vi "Pomiar_UceIc.vi"(0 "Komutator L201":refnum<visa-resource-name>, 1 "Zasilacz BM572":refnum<visa-resource-name>, 2 "STOP":refnum<vi>, 5 "Samples":dbl[](array[numeric]), 9 "Multimetr V553":refnum<visa-resource-name>, 11 "Maksymalna moc tranzystora":dbl) -> (3 "Uce":dbl[](array[numeric]), 4 "Ic":dbl[](array[numeric]), 6 "Komutator L201 out":refnum<visa-resource-name>, 10 "Moc [W]":dbl[](array[numeric]), 12 "Multimetr V553 out":refnum<visa-resource-name>, 14 "Zasilacz BM572 out":refnum<visa-resource-name>, 15 "Index":i32)   [LabVIEW 2023]
panel:
  out "element":dbl
  out "String":string
  out "error constant 3":errorcluster
  out "error constant 2":errorcluster
  out "error constant":errorcluster
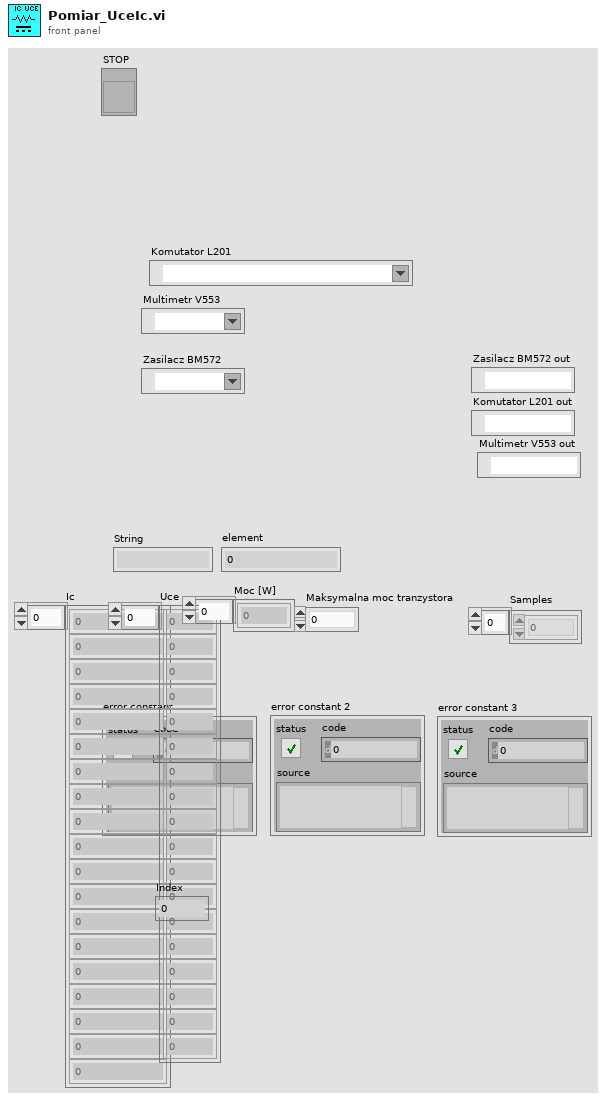
[diagram p1: front panel]
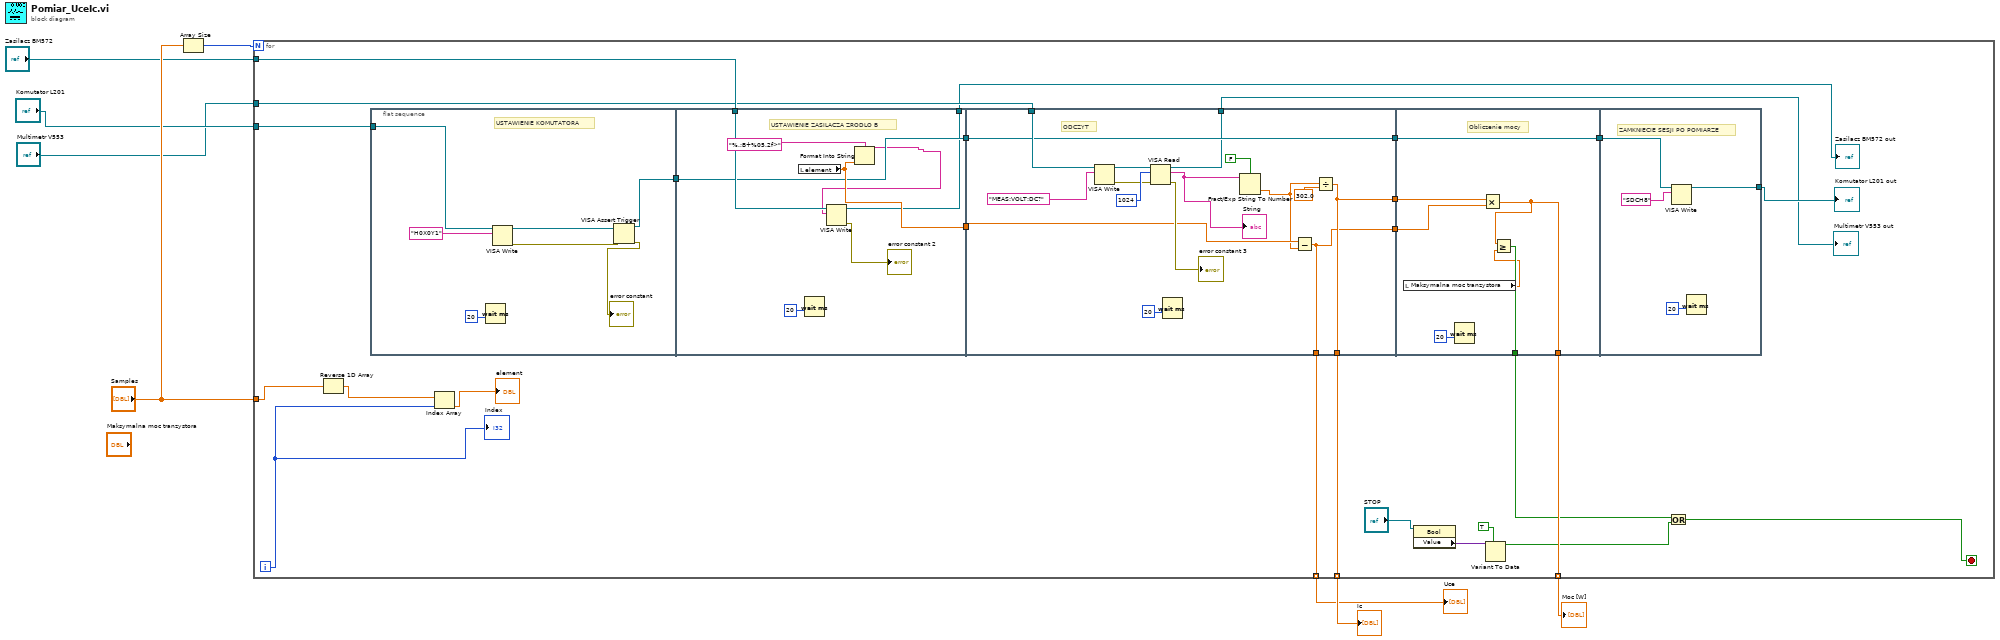
[diagram p0: block diagram]
diagram:
  n1 = Array Size(array="Samples") -> (size(s)=w8:i32)
  n2 = for {
    N: w8 -> [_]
    tunnel: "Samples" -> [w19]
    tunnel: "Komutator L201" -> [w29]
    tunnel: "Zasilacz BM572" -> [w28]
    tunnel: "Multimetr V553" -> [w27]
    tunnel: [w17] -> w3 mode=indexing
    tunnel: [w16] -> w2 mode=indexing
    tunnel: [w15] -> w1 mode=indexing
    i -> [w30]
    stop <- w13 stop-if-true
    n3 = Reverse 1D Array(array=w19) -> (reversed array=w18:dbl[])
    n4 = flat-sequence {
      tunnel: w29 -> [w36]
      tunnel: [w35] -> w23
      tunnel: [w46] -> w31
      tunnel: w28 -> [w45]
      tunnel: [w44] -> w24
      tunnel: w23 -> [w44]
      tunnel: [w43] -> w20
      tunnel: [w54] -> w34
      tunnel: [w53] -> w33
      tunnel: w31 -> [w58]
      tunnel: w27 -> [w57]
      tunnel: [w56] -> w25
      tunnel: w24 -> [w56]
      tunnel: [w55] -> w21
      tunnel: [w54] -> w17
      tunnel: [w53] -> w16
      tunnel: w34 -> [w72]
      tunnel: w33 -> [w71]
      tunnel: [w69] -> w14
      tunnel: [w67] -> w26
      tunnel: w25 -> [w67]
      tunnel: [w66] -> w15
      tunnel: w26 -> [w74]
      tunnel: [w73] -> w22
      frame #0 {
        # "USTAWIENIE KOMUTATORA"
        n5 = Wait (ms)(milliseconds to wait=u32 20) -> ()  [unwired: 1 out]
        n6 = VISA Write(VISA resource name=w36, write buffer="H0X0Y1") -> (VISA resource name out=w37:refnum<visa-resource-name>, error out=w39:errorcluster)  [unwired: 1 in, 1 out]
        n7 = VISA Assert Trigger(8:w39, 11:w37) -> (0:→"error constant":errorcluster, 3:w35:refnum<visa-resource-name>)  [unwired: 1 in]
      }
      frame #1 {
        # "USTAWIENIE ZASILACZA ZRODLO B"
        n8 = local read "element"() -> (w46:dbl)
        n9 = Wait (ms)(milliseconds to wait=u32 20) -> ()  [unwired: 1 out]
        n10 = Format Into String(format string="%.;B+%05.2f>", w46) -> (resulting string=w42:string)  [unwired: 2 in, 1 out]
        n11 = VISA Write(VISA resource name=w45, write buffer=w42) -> (VISA resource name out=w43:refnum<visa-resource-name>, error out=→"error constant 2":errorcluster)  [unwired: 1 in, 1 out]
      }
      frame #2 {
        # "ODCZYT"
        n12 = VISA Write(VISA resource name=w57, write buffer="MEAS:VOLT:DC?") -> (VISA resource name out=w63:refnum<visa-resource-name>, error out=w62:errorcluster)  [unwired: 1 in, 1 out]
        n13 = VISA Read(VISA resource name=w63, byte count=u32 1024, error in (no error)=w62) -> (VISA resource name out=w55:refnum<visa-resource-name>, read buffer=w52:string, error out=→"error constant 3":errorcluster)  [unwired: 1 out]
        "String" <- w52
        n14 = Wait (ms)(milliseconds to wait=u32 20) -> ()  [unwired: 1 out]
        n15 = Fract/Exp String To Number(use system decimal point (T)=FALSE, string=w52) -> (number=w51:dbl)  [unwired: 2 in, 1 out]
        n16 = Subtract(x=w58, y=w51) -> (x-y=w53:dbl)
        n17 = Divide(x=w51, y=302.0) -> (x/y=w54:dbl)
      }
      frame #3 {
        # "Obliczenie mocy"
        n18 = local read "Maksymalna moc tranzystora"() -> (w68:dbl)
        n19 = Wait (ms)(milliseconds to wait=u32 20) -> ()  [unwired: 1 out]
        n20 = Multiply(x=w72, y=w71) -> (x*y=w66:dbl)
        n21 = Greater Or Equal?(x=w66, y=w68) -> (x >= y?=w69:bool)
      }
      frame #4 {
        # "ZAMKNIECIE SESJI PO POMIARZE"
        n22 = VISA Write(VISA resource name=w74, write buffer="SDCH8") -> (VISA resource name out=w73:refnum<visa-resource-name>)  [unwired: 1 in, 2 out]
        n23 = Wait (ms)(milliseconds to wait=u32 20) -> ()  [unwired: 1 out]
      }
    }
    n24 = Index Array(array=w18, index=w30) -> (element=→"element":dbl)
    n25 = property class="Bool"(reference="STOP") -> ("Value"=w11:variant)  [unwired: 1 in, 2 out]
    n26 = Variant To Data(type=TRUE, Variant=w11) -> (data=w9:bool)  [unwired: 1 in, 1 out]
    n27 = Or(x=w14, y=w9) -> (x .or. y?=w13:bool)
    "Index" <- w30
    "Zasilacz BM572 out" <- w20
    "Komutator L201 out" <- w22
    "Multimetr V553 out" <- w21
  }
  "Ic" <- w3
  "Uce" <- w2
  "Moc [W]" <- w1
